vi "Config Voltage.vi"(8 "error in":errorcluster, 10 "Voltage (15 V)":dbl=15.0 min=0.0003 max=15.0 step=1.0 format="%#.6f", 11 "VISA resource name":refnum<visa-resource-name>) -> (0 "error out":errorcluster, 3 "VISA resource name out":refnum<visa-resource-name>)   [LabVIEW 2025]
doc: "This VI limits the amplitude of the AC RMS voltage applied by the bridge to the device under test."
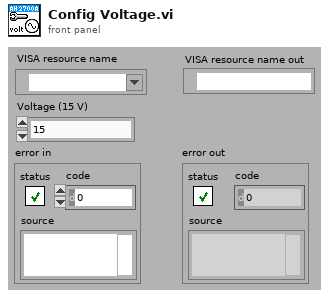
[diagram p1: front panel]
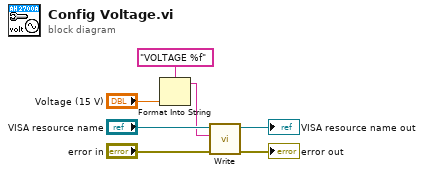
[diagram p0: block diagram]
diagram:
  n1 = Format Into String(format string="VOLTAGE %f", "Voltage (15 V)") -> (resulting string=w6:string)  [unwired: 2 in, 1 out]
  n2 = call "Write.vi"("error in"="error in", "command"=w6, "VISA resource name"="VISA resource name") -> ("error out"=→"error out":errorcluster, "VISA resource name out"=→"VISA resource name out":refnum<visa-resource-name>)  [unwired: 7 in]
